vi "ProcessingData.vi"(5 "Output Values of Device":refnum<vi>, 9 "Main menu in":refnum<vi>, 10 "KEITHLEY 2182 & KEITHLEY 6222":refnum<vi>, 11 "Cluster in":refnum<vi>) -> (1 "Main menu out":refnum<vi>, 2 "KEITHLEY 2182 & KEITHLEY 6221":refnum<vi>, 3 "Cluster out":refnum<vi>)   [LabVIEW 2013]
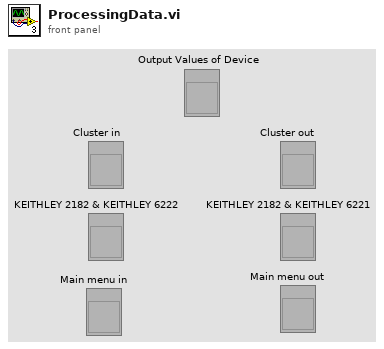
[diagram p1: front panel]
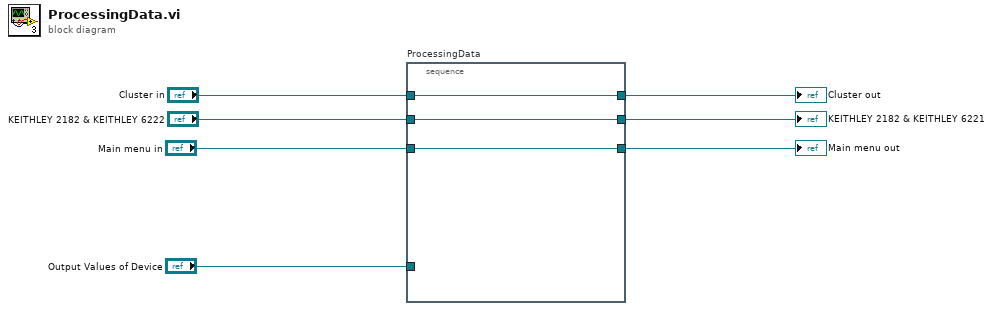
[diagram p0: block diagram]
diagram:
  n1 = stacked-sequence "ProcessingData" {
    tunnel: "KEITHLEY 2182 & KEITHLEY 6222" -> [w10]
    tunnel: "Main menu in" -> [w9]
    tunnel: [w10] -> w4
    tunnel: [w9] -> w5
    tunnel: [w8] -> w7
    tunnel: "Cluster in" -> [w8]
    tunnel: "Output Values of Device" -> [_]
    frame #0 {
    }
  }
  "Cluster out" <- w7
  "Main menu out" <- w5
  "KEITHLEY 2182 & KEITHLEY 6221" <- w4
